vi "BuildByteWithParity_no HW compare.vi"(6 "Parity Count In":u8, 7 "Read/Write Data":T3 {"Data" format="%.0x"}, 8 "error in":errorcluster, 9 "Number of Samples In":i32, 10 "Data Array In":u8[][](array[numeric]), 11 "RFFE_Data In":T1 {"Toggle (high to low)" items=["0", "1", "Z", "L", "H", "X", "T", "V"]; "X Array" items=["0", "1", "Z", "L", "H", "X", "T", "V"]; "Z Array" items=["0", "1", "Z", "L", "H", "X", "T", "V"]; "L Array" items=["0", "1", "Z", "L", "H", "X", "T", "V"]; "H Array" items=["0", "1", "Z", "L", "H", "X", "T", "V"]; "One Array" items=["0", "1", "Z", "L", "H", "X", "T", "V"]; "Zero Array" items=["0", "1", "Z", "L", "H", "X", "T", "V"]}) -> (0 "error out":errorcluster, 1 "Number of Samples Out":i32, 2 "Data Array Out":u8[][](array[numeric]), 3 "RFFE_Data Out":T1 {"Toggle (high to low)" items=["0", "1", "Z", "L", "H", "X", "T", "V"]; "X Array" items=["0", "1", "Z", "L", "H", "X", "T", "V"]; "Z Array" items=["0", "1", "Z", "L", "H", "X", "T", "V"]; "L Array" items=["0", "1", "Z", "L", "H", "X", "T", "V"]; "H Array" items=["0", "1", "Z", "L", "H", "X", "T", "V"]; "One Array" items=["0", "1", "Z", "L", "H", "X", "T", "V"]; "Zero Array" items=["0", "1", "Z", "L", "H", "X", "T", "V"]}, 5 "Compare Locations":u32[](array[numeric]))   [LabVIEW 2013]
doc: "Builds byte with optional parity bit."
uses:
  Ctrls/RFFE_Data.ctl
  Ctrls/ClockDataChannels.ctl
  Ctrls/Read_Write_Data.ctl
  Ctrls/BitStates.ctl
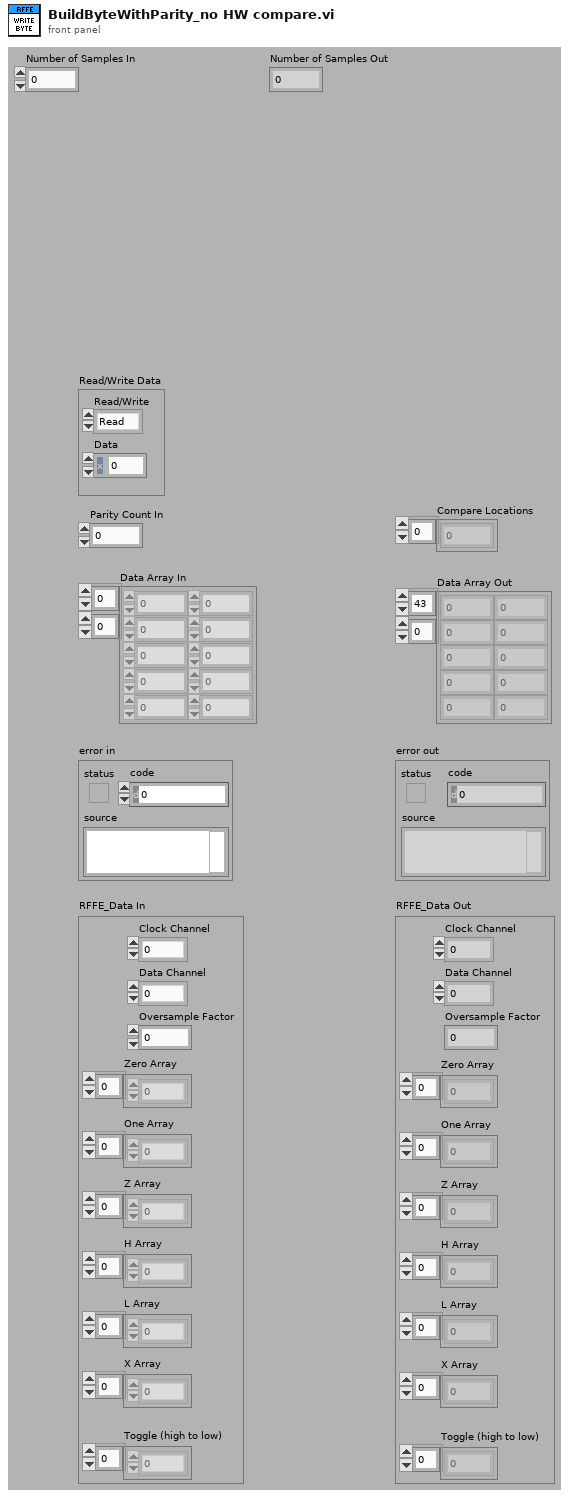
[diagram p1: front panel]
types:
  T1 = typedef "RFFE_Data.ctl" = cluster{"Clock Channel":T2, "Data Channel":T2, "Oversample Factor":u8, "Zero Array":u8[], "One Array":u8[], "Z Array ":u8[], "H Array":u8[], "L Array":u8[], "X Array":u8[], "Toggle (high to low)":u8[]}
  T2 = typedef "ClockDataChannels.ctl" = enum16{"0", "1"}
  T3 = typedef "Read_Write_Data.ctl" = cluster{"Data":u8, "Read/Write":enum16{"Read", "Write"}}
  T4 = typedef "BitStates.ctl" = enum16{"0", "1", "Z", "L", "H", "X", "Toggle"}
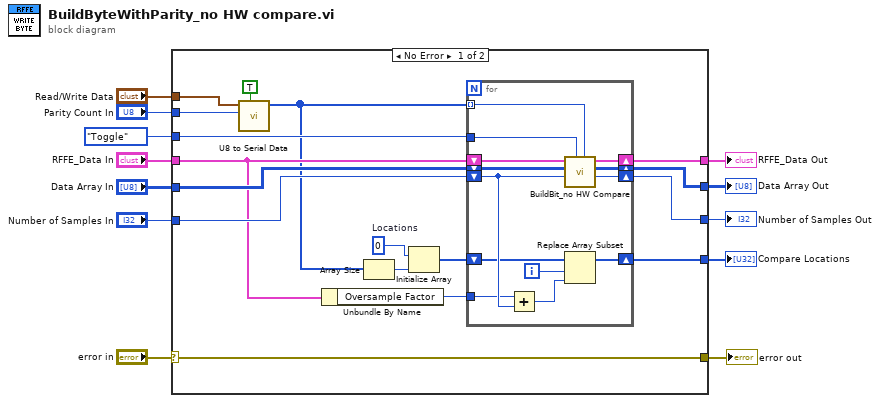
[diagram p0: block diagram]
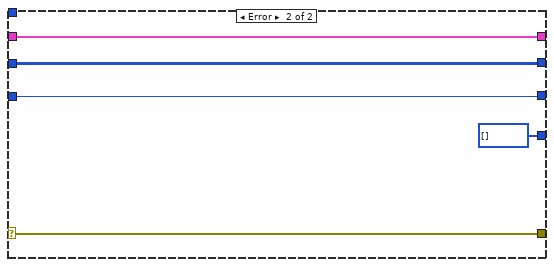
[diagram p2: hidden frame]
diagram:
  n1 = case shown="No Error" "error in" {
    selector: "error in" -> [w13 w47]
    tunnel: BitStates."Toggle" ("Data Value") -> [w29 _]
    tunnel: "Parity Count In" -> [w28 _]
    tunnel: [w26 w44] -> w10
    tunnel: [w25 w45] -> w9
    tunnel: "Data Array In" -> [w24 w45]
    tunnel: "Number of Samples In" -> [w23 w44]
    tunnel: [w22 w46] -> w6
    tunnel: "RFFE_Data In" -> [w21 w46]
    tunnel: "Read/Write Data" -> [w19 _]
    tunnel: [w14 u32[] []] -> w3
    tunnel: [w13 w47] -> w1
    frame No Error {
      w18 = u32 0  # Locations
      n2 = call "U8 to Serial Data.vi"("Parity Bit?"=TRUE, "Parity Count In"=w28, "Read/Write Data"=w19) -> ("Data Values"=w15:T4[])  [unwired: 7 in, 1 out]
      n3 = Unbundle By Name(w21) -> ("Oversample Factor"=w20:u8)
      n4 = Array Size(array=w15) -> (size(s)=w17:i32)
      n5 = Initialize Array(w18, w17) -> (w16:u32[])
      n6 = for {
        tunnel: w29 -> [w40]
        shift-right: [w38] -> w25
        shift-left: w24 -> [w42]
        shift-right: [w37] -> w22
        shift-left: w21 -> [w41]
        shift-right: [w39] -> w26
        shift-left: w23 -> [w34]
        tunnel: w15 -> [w36] mode=indexing
        shift-right: [w35] -> w14
        shift-left: w16 -> [w31]
        tunnel: w20 -> [w33]
        i -> [w32]
        n7 = Add(x=w33, y=w34) -> (x+y=w30:i32)
        n8 = call "BuildBit_no HW Compare.vi"("Data Value"=w36, "Clock Value"=w40, "Number of Samples In"=w34, "Data Array In"=w42, "RFFE_Data In"=w41) -> ("Number of Samples Out"=w39:i32, "Data Array Out"=w38:u8[][], "RFFE_Data Out"=w37:T1)  [unwired: 4 in]
        n9 = Replace Array Subset(array=w31, new element=w30, index=w32) -> (w35:u32[])
      }
    }
    frame Error {
    }
  }
  "Data Array Out" <- w9
  "Number of Samples Out" <- w10
  "error out" <- w1
  "RFFE_Data Out" <- w6
  "Compare Locations" <- w3
